vi "getEnabledChannels.vi"(6 "Enable":bool, 8 "error in (no error)":errorcluster, 9 "Channel (0.1.2.3)":string, 11 "Refnum in":refnum<k21>) -> (0 "error out":errorcluster, 1 "Channels":refnum<k21>[](array[refnum]), 2 "Enable (Array)":bool[](array[boolean]), 3 "Refnum out":refnum<k21>)   [LabVIEW 2011]
uses:
  C:/Program Files/National Instruments/LabVIEW 2011/resource/objmgr/daqmx.rc
panel:
  out "Numeric":i32
  in  "Channels 2":refnum<k21>[](array[refnum])
  in  "Array":tag[](array[tag])
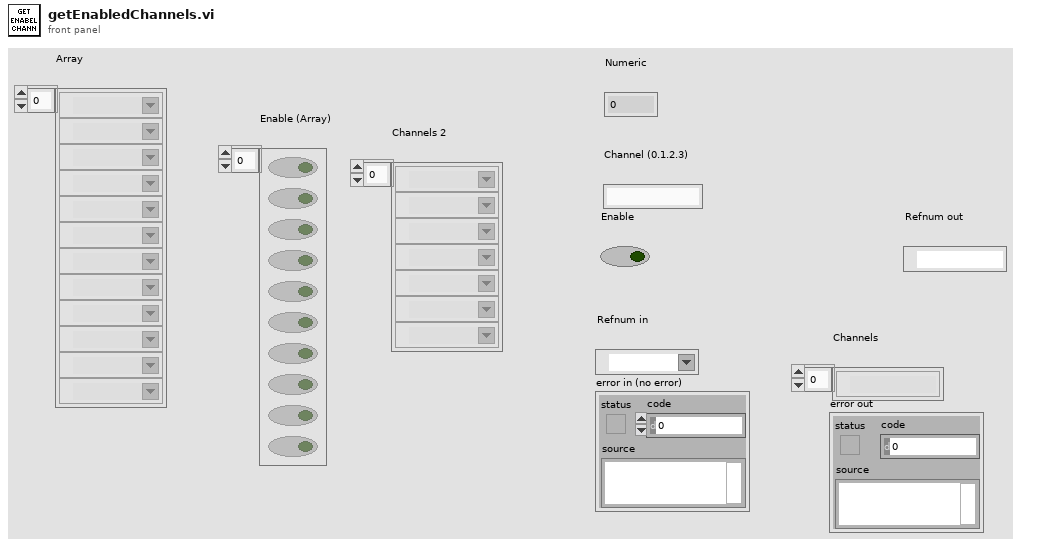
[diagram p1: front panel]
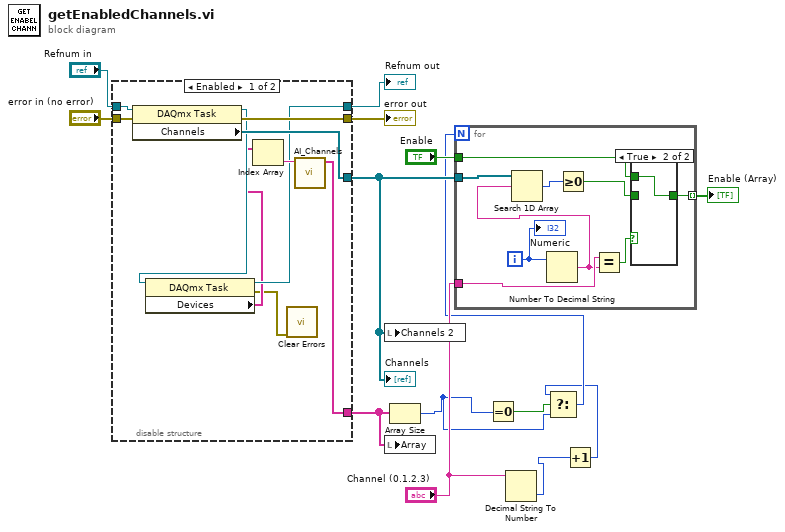
[diagram p0: block diagram]
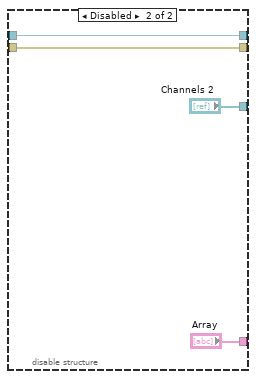
[diagram p2: hidden frame]
diagram:
  n1 = disable-structure shown="Enabled" {
    disable-tunnel: "Refnum in" -> [w24 w27]
    disable-tunnel: [w17 w27] -> w12
    disable-tunnel: "error in (no error)" -> [w23 w26]
    disable-tunnel: [w22 w26] -> w10
    disable-tunnel: [w20 "Channels 2"] -> w8
    disable-tunnel: [w19 "Array"] -> w7
    frame Enabled {
      n2 = property class="DAQmx Task"(reference=w24, error in=w23) -> (reference out=w18:refnum<k21>, error out=w22:errorcluster, "Channels"=w20:refnum<k21>[])
      n3 = property class="DAQmx Task"(reference=w18) -> (reference out=w17:refnum<k21>, error out=w15:errorcluster, "Devices"=w16:tag[])  [unwired: 1 in]
      n4 = Index Array(array=w16) -> (element=w21:tag)  [unwired: 1 in]
      n5 = call "Clear Errors.vi"("error in (no error)"=w15) -> ()  [unwired: 6 in, 1 out]
      n6 = call "AI_Channels.vi"("DAQmx Device Name"=w21) -> ("Array"=w19:tag[])  [unwired: 9 in, 1 out]
    }
    frame Disabled {
    }
  }
  "Channels" <- w8
  "Refnum out" <- w12
  "error out" <- w10
  n7 = local write "Channels 2"(w8) -> ()
  n8 = local write "Array"(w7) -> ()
  n9 = Array Size(array=w7) -> (size(s)=w4:i32)
  n10 = Equal To 0?(x=w4) -> (x = 0?=w5:bool)
  n11 = Decimal String To Number(string="Channel (0.1.2.3)") -> (number=w2:i32)  [unwired: 2 in, 1 out]
  n12 = Increment(x=w2) -> (x+1=w1:i32)
  n13 = Select(t=w1, s=w5, f=w4) -> (s? t:f=w3:i32)
  n14 = for {
    N: w3 -> [_]
    tunnel: [w34] -> w14 mode=indexing
    tunnel: "Enable" -> [w35]
    tunnel: "Channel (0.1.2.3)" -> [w37]
    tunnel: w8 -> [w32]
    i -> [w33]
    n15 = Number To Decimal String(number=w33) -> (decimal integer string=w31:string)  [unwired: 1 in]
    n16 = Search 1D Array(1D array=w32, element=w31) -> (index of element=w30:i32)  [unwired: 1 in]
    n17 = Greater Or Equal To 0?(x=w30) -> (x >= 0?=w29:bool)
    n18 = Equal?(x=w37, y=w31) -> (x = y?=w36:bool)
    n19 = case shown="True" w36 {
      tunnel: w35 -> [_ w39]
      tunnel: [w38 w39] -> w34
      tunnel: w29 -> [w38 _]
      frame False {
      }
      frame True {
      }
    }
    "Numeric" <- w33
  }
  "Enable (Array)" <- w14
